vi "Write 7z bat.vi"(8 "error in (no error)":errorcluster, 11 "PostBuildSupport in":refnum<class "PostBuildSupport.lvclass">) -> (0 "error out":errorcluster, 3 "PostBuildSupport out":refnum<class "PostBuildSupport.lvclass">)   [LabVIEW 2016, in "PostBuildSupport.lvclass"]
uses:
  PostBuildSupport.lvclass
  PostBuildSupport.lvclass/PostBuildSupport.ctl
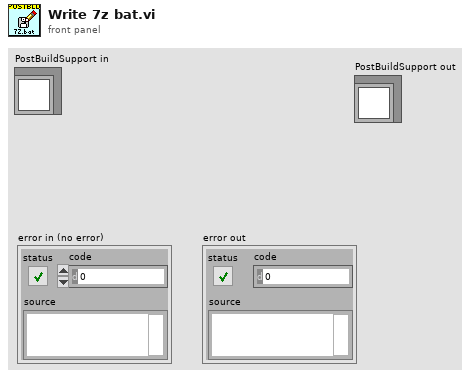
[diagram p1: front panel]
types:
  T1 = enum16{"open", "replace", "create", "open or create", "replace or create", "replace or create with confirmation"}
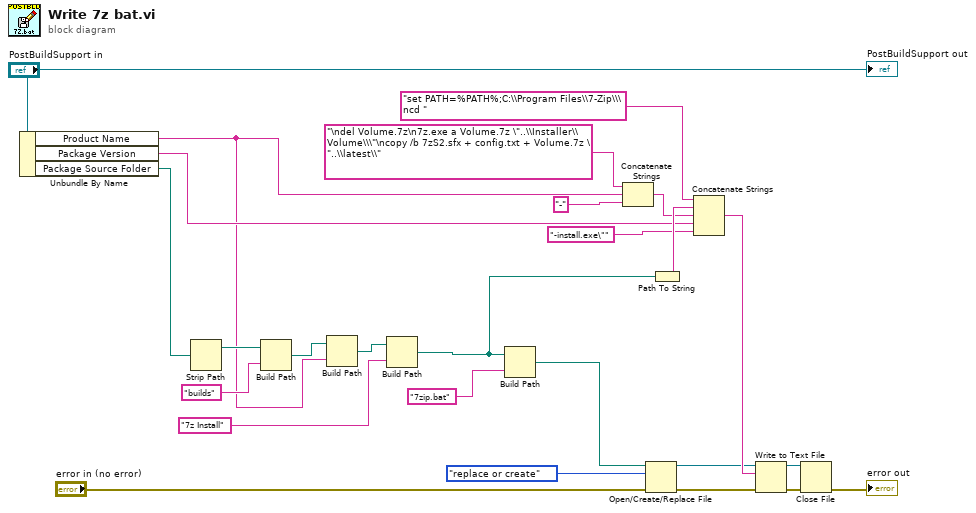
[diagram p0: block diagram]
diagram:
  n1 = Unbundle By Name("PostBuildSupport in") -> ("Product Name"=w4:string, "Package Version"=w8:string, "Package Source Folder"=w7:path)
  n2 = Strip Path(path=w7) -> (stripped path=w23:path)  [unwired: 1 out]
  n3 = Build Path(base path=w23, name or relative path="builds") -> (appended path=w5:path)
  n4 = Build Path(base path=w5, name or relative path=w4) -> (appended path=w3:path)
  n5 = Build Path(base path=w3, name or relative path="7z Install") -> (appended path=w1:path)
  n6 = Build Path(base path=w1, name or relative path="7zip.bat") -> (appended path=w21:path)
  n7 = Concatenate Strings("\ndel Volume.7z\n7z.exe a Volume.7z \"..\\Installer\\Volume\\\"\ncopy /b 7zS2.sfx + config.txt + Volume.7z \"..\\latest\\" ("Name of target (My Computer)"), w4, "-" ("Name of target (My Computer)")) -> (w11:string)
  n8 = Open/Create/Replace File(file path (use dialog)=w21, error in="error in (no error)", operation (0:open)=T1."replace or create") -> (refnum out=w22:refnum<file>, error out=w19:errorcluster)  [unwired: 3 in, 1 out]
  n9 = Path To String(path=w1) -> (string=w14:string)
  n10 = Concatenate Strings("set PATH=%PATH%;C:\\Program Files\\7-Zip\\\ncd " ("Name of target (My Computer)"), w14, w11, w8, "-install.exe\"" ("Name of target (My Computer)")) -> (w26:string)
  n11 = Write to Text File(file (use dialog)=w22, text=w26, error in=w19) -> (refnum out=w16:refnum<file>, error out=w17:errorcluster)  [unwired: 1 in, 1 out]
  n12 = Close File(refnum=w16, error in=w17) -> (error out=→"error out":errorcluster)  [unwired: 1 out]
  "PostBuildSupport out" <- "PostBuildSupport in"
